vi "mW_EIP_Read.vi"(7 "error in (no error)":errorcluster, 10 "VISA Refnum in":refnum<visa-resource-name>) -> (0 "error out":errorcluster, 1 "No Reading":bool, 2 "Frequency":dbl, 3 "VISA resource name out":refnum<visa-resource-name>)   [LabVIEW 2019]
uses:
  <vilib>/Analysis/baseanly.llb/Mean (DBL).vi
  <vilib>/Analysis/NI_AALBase.lvlib
panel:
  out "Error":bool
  out "iterations":i32
  in  "n_samples":i32=10
  out "Array":dbl[](array[numeric])
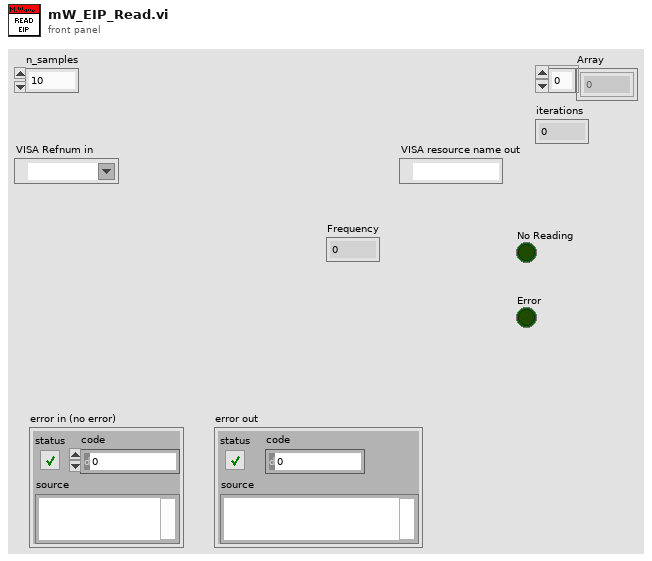
[diagram p1: front panel]
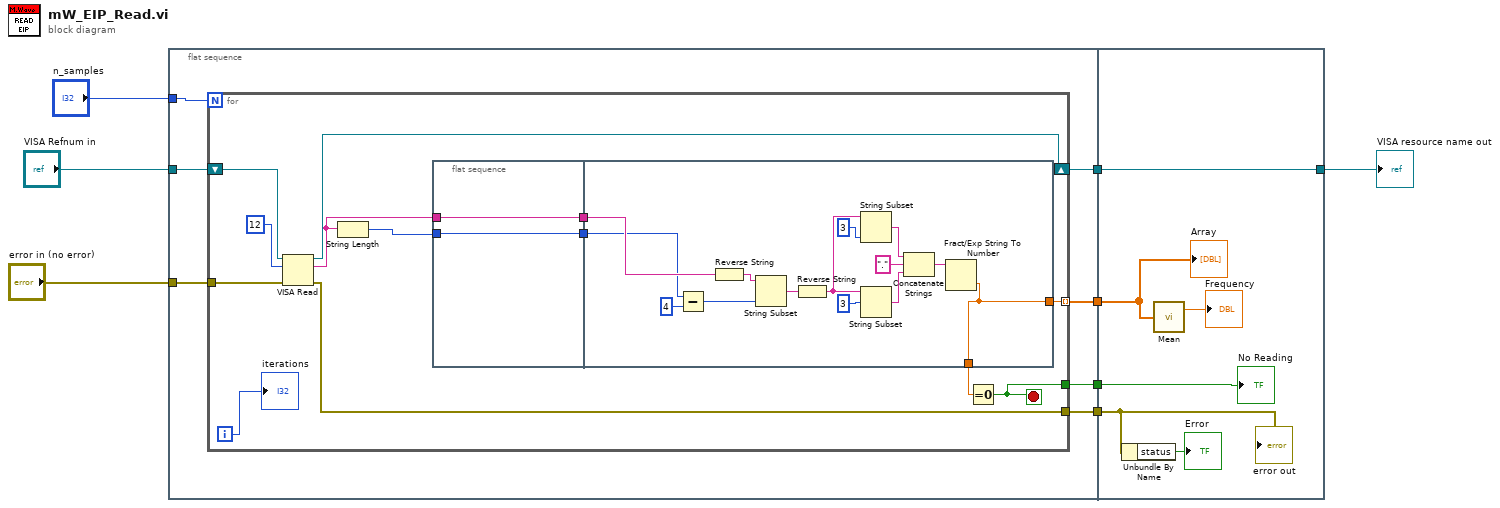
[diagram p0: block diagram]
diagram:
  n1 = flat-sequence {
    tunnel: "error in (no error)" -> [w15]
    tunnel: "VISA Refnum in" -> [w14]
    tunnel: "n_samples" -> [w12]
    tunnel: [w13] -> w4
    tunnel: [w11] -> w3
    tunnel: [w10] -> w2
    tunnel: [w9] -> w1
    tunnel: [w50] -> w6
    tunnel: w4 -> [w50]
    tunnel: w3 -> [w48]
    tunnel: w2 -> [w47]
    tunnel: w1 -> [w45]
    frame #0 {
      n2 = for {
        N: w12 -> [_]
        tunnel: w15 -> [w28]
        shift-right: [w24] -> w13
        shift-left: w14 -> [w25]
        tunnel: [w23] -> w11 mode=indexing
        tunnel: [w22] -> w10
        tunnel: [w16] -> w9
        i -> [w19]
        stop <- w16 stop-if-true
        n3 = VISA Read(VISA resource name=w25, byte count=u32 12, error in (no error)=w28) -> (VISA resource name out=w24:refnum<visa-resource-name>, read buffer=w26:string, error out=w22:errorcluster)  [unwired: 1 out]
        n4 = String Length(string=w26) -> (length=w18:i32)
        n5 = flat-sequence {
          tunnel: w18 -> [w29]
          tunnel: w26 -> [w30]
          tunnel: [w30] -> w21
          tunnel: [w29] -> w20
          tunnel: [w31] -> w23
          tunnel: w21 -> [w44]
          tunnel: w20 -> [w43]
          tunnel: [w31] -> w17
          frame #0 {
          }
          frame #1 {
            n6 = Subtract(x=w43, y=4) -> (x-y=w40:i32)
            n7 = Reverse String(1:w44) -> (0:w41:string)
            n8 = String Subset(string=w41, length (rest)=w40) -> (substring=w39:string)  [unwired: 1 in]
            n9 = Reverse String(1:w39) -> (0:w37:string)
            n10 = String Subset(string=w37, length (rest)=3 ("length (rest)")) -> (substring=w34:string)  [unwired: 1 in]
            n11 = String Subset(string=w37, offset (0)=3) -> (substring=w35:string)  [unwired: 1 in]
            n12 = Concatenate Strings(w34, "." ("string"), w35) -> (w32:string)
            n13 = Fract/Exp String To Number(string=w32) -> (number=w31:dbl)  [unwired: 3 in, 1 out]
          }
        }
        n14 = Equal To 0?(x=w17) -> (x = 0?=w16:bool)
        "iterations" <- w19
      }
    }
    frame #1 {
      n15 = Unbundle By Name(w47) -> ("status"=→"Error":bool)
      n16 = call-poly <vilib>:"Mean.vi"("X"=w48) -> ("mean"=→"Frequency":dbl)  [unwired: 1 out]
      "Array" <- w48
      "error out" <- w47
      "No Reading" <- w45
    }
  }
  "VISA resource name out" <- w6
